vi "List columns.vi"(8 "error in (no error)":errorcluster, 9 "显示关键参数":bool, 10 "table":string, 11 "database":string="database1.mdb") -> (0 "error out":errorcluster, 3 "columns":string[](array[string]))   [LabVIEW 2016, in "数据查询.lvlib"]
uses:
  <vilib>/addons/database/Connection.llb/DB Tools Open Connec (String).vi
  <userlib>/_LVST/sqlite_api/Core/Tables/SQLite_List Columns.vi
  <userlib>/_OpenG.lib/array/array.llb/Filter 1D Array (String)__ogtk.vi
  <vilib>/addons/database/NI_Database_API.lvlib
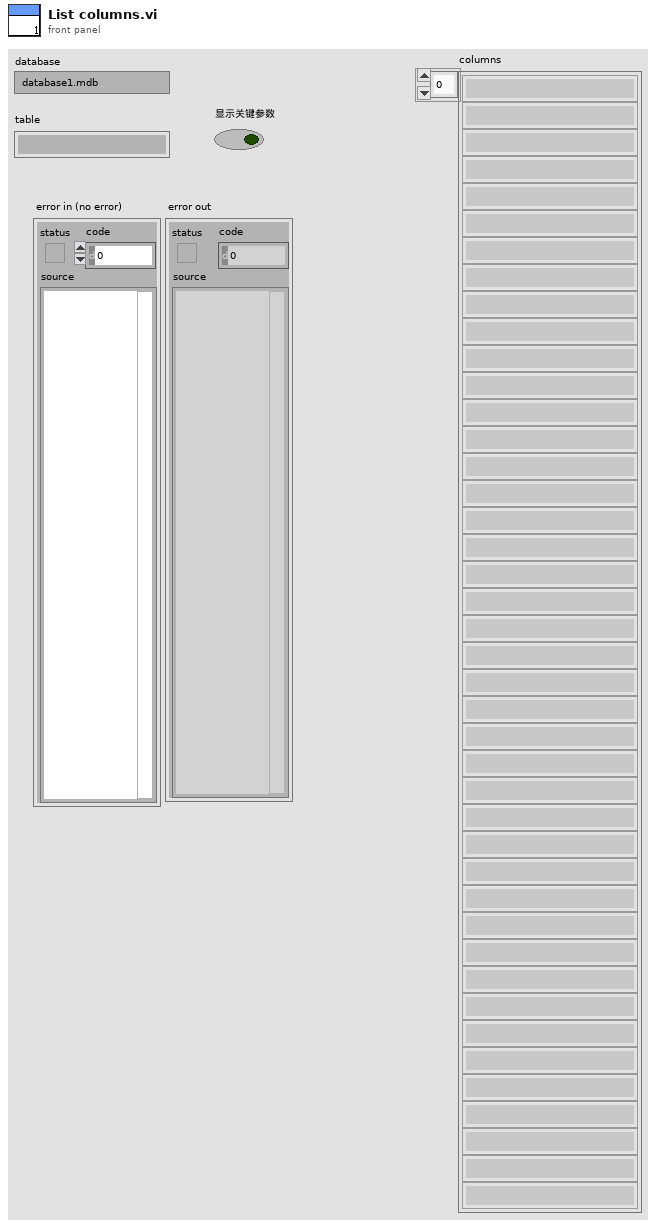
[diagram p1: front panel]
types:
  T1 = typedef "数据库类型.ctl" = enum16{"Access", "SQLite"}
  T2 = typedef "NI_Database_API.lvlib/Conn ObjectReference.ctl" = refnum<k1>
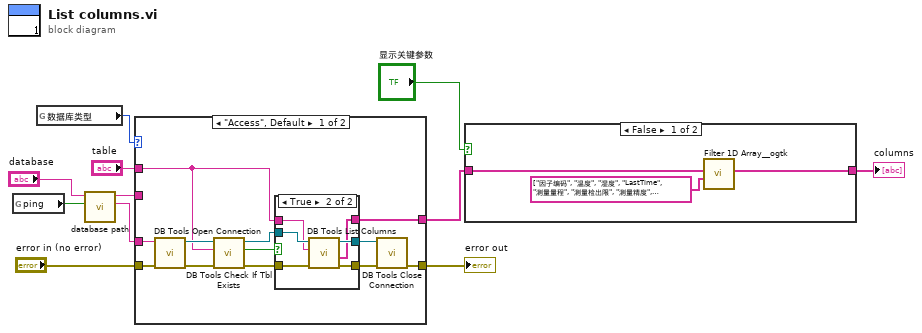
[diagram p0: block diagram]
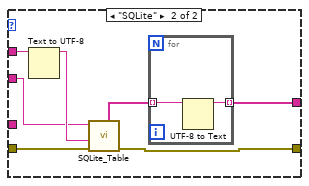
[diagram p4: hidden frame]
diagram:
  n1 = global read "全局变量.vi" "ping"() -> (w6:bool)
  n2 = global read "外部调用接口全局变量.vi" "数据库类型"() -> (w1:T1)
  n3 = call "database path.vi"("ping"=w6, "database"="database") -> ("Connection information"=w2:string, "Path out"=w7:string)  [unwired: 8 in]
  n4 = case shown="\"Access\", Default" w1 {
    tunnel: "table" -> [w14 w34]
    tunnel: "error in (no error)" -> [w21 w37]
    tunnel: [w20 w38] -> w9
    tunnel: [w19 w35] -> w4
    tunnel: w7 -> [_ w32]
    tunnel: w2 -> [w18 _]
    frame "Access", Default {
      n5 = call-poly <vilib>:"DB Tools Open Connection.vi"("error in (no error)"=w21, "connection information"=w18) -> ("error out"=w15:errorcluster, "connection reference"=w17:T2)  [unwired: 6 in]
      n6 = call <vilib>:"DB Tools Check If Tbl Exists.vi"("error in (no error)"=w15, "table name"=w14, "connection reference"=w17) -> ("error out"=w13:errorcluster, "exists?"=w12:bool, "connection reference out"=w16:T2)  [unwired: 2 out]
      n7 = case shown="True" w12 {
        tunnel: [w25 w31] -> w23
        tunnel: [w24 w30] -> w22
        tunnel: [_ w29] -> w19
        tunnel: w16 -> [w25 w28]
        tunnel: w14 -> [_ w27]
        tunnel: w13 -> [w24 w26]
        frame False {
        }
        frame True {
          n8 = call <vilib>:"DB Tools List Columns.vi"("error in (no error)"=w26, "table"=w27, "connection reference"=w28) -> ("error out"=w30:errorcluster, "columns"=w29:string[], "connection reference out"=w31:T2)  [unwired: 1 in, 1 out]
        }
      }
      n9 = call <vilib>:"DB Tools Close Connection.vi"("error in (no error)"=w22, "connection reference"=w23) -> ("error out"=w20:errorcluster)  [unwired: 5 in]
    }
    frame "SQLite" {
      n10 = Text to UTF-8(11:w34) -> (3:w33:string)  [unwired: 2 in, 1 out]
      n11 = call-poly <userlib>:"SQLite_Table.vi"("DB Path"=w32, "Table Name"=w33, "error in (no error)"=w37) -> ("Columns"=w36:string[], "error out"=w38:errorcluster)  [unwired: 4 in, 2 out]
      n12 = for {
        tunnel: w36 -> [w40] mode=indexing
        tunnel: [w39] -> w35 mode=indexing
        n13 = UTF-8 to Text(11:w40) -> (3:w39:string)  [unwired: 2 in, 1 out]
      }
    }
  }
  "error out" <- w9
  n14 = case shown="False" "显示关键参数" {
    tunnel: w4 -> [w43 w44]
    tunnel: [w41 w44] -> w3
    frame False {
      n15 = call-poly <userlib>:"Filter 1D Array__ogtk.vi"("items to filter"=string[] ["因子编码", "温度", "湿度", "LastTime", "测量量程", "测量检出限", "测量精度", "测量间隔", "消解温度", "消解时长", "三项式系数", "二次多项式系数", "曲线斜率", "曲线截距", "线性相关系数", "空白校准时间", "标样校准时间", "测量信号值", "稀释倍数", "空白标定系数", "量程系数", "X1"] ("columns"), "array"=w43) -> ("filtered array"=w41:string[])  [unwired: 4 in, 1 out]
    }
    frame True {
    }
  }
  "columns" <- w3
